vi "_Enqueue JKISMQ.vi"(8 "Error in":errorcluster caption="Error in (no error)", 10 "Data":T1, 11 "JKISMQ":T2) -> (0 "Error out":errorcluster, 3 "JKISMQ":T2)   [LabVIEW 2020, in "JKI-State-Machine-Plus.lvlib"]
uses:
  JKI-State-Machine-Plus.lvlib
  _JKISMQ.ctl
  _Cross JKI StateMachine State Data.ctl
  _Cross JKI StateMachine State Response.ctl
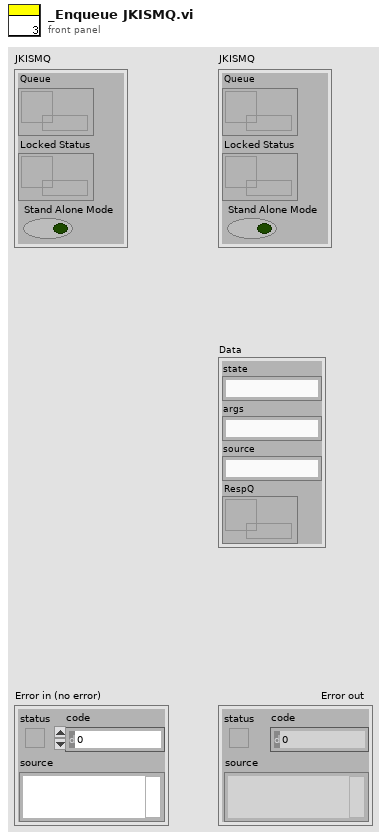
[diagram p1: front panel]
types:
  T1 = typedef "JKI-State-Machine-Plus.lvlib/_Cross JKI StateMachine State Data.ctl" = cluster{"state":string, "args":string, "source":string, "RespQ":refnum<queue>}
  T2 = typedef "JKI-State-Machine-Plus.lvlib/_JKISMQ.ctl" = cluster{"Queue":refnum<queue>, "Locked Status":refnum<data-value>, "Stand Alone Mode":bool}
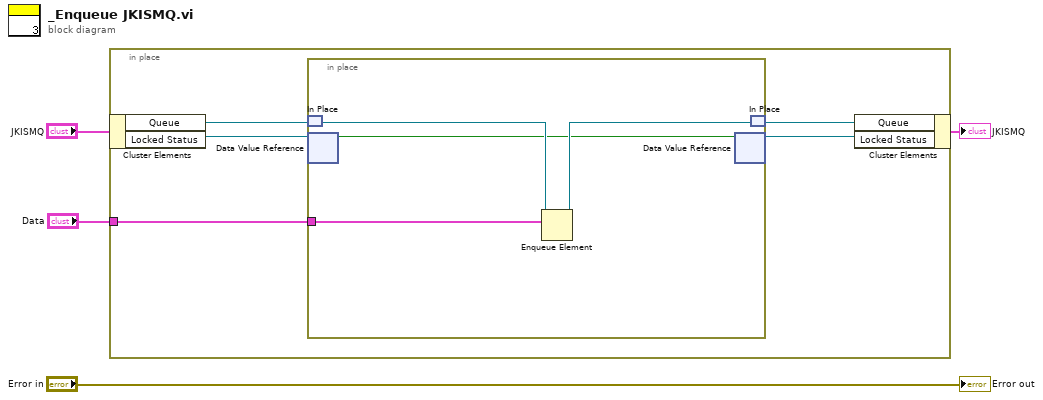
[diagram p0: block diagram]
diagram:
  n1 = in-place "In Place Element Structure" {
    in-place-border: "Data" -> [w5]
    n2 = in-place-cluster #1("JKISMQ") -> ("Queue"=w9:refnum<queue>, "Locked Status"=w7:refnum<data-value>)
    n3 = in-place {
      in-place-border: w5 -> [w10]
      n4 = in-place-match #2(w9) -> (w12:refnum<queue>)
      n5 = in-place-dvr #3(w7) -> (w11:bool)  [unwired: 1 out]
      n6 = Enqueue Element(queue=w12, element=w10) -> (queue out=w13:refnum<queue>)  [unwired: 2 in, 2 out]
      n7 = in-place-dvr #3(w11) -> (w6:refnum<data-value>)  [unwired: 1 out]
      n8 = in-place-match #2(w13) -> (w8:refnum<queue>)
    }
    n9 = in-place-cluster #1("Queue"=w8, "Locked Status"=w6) -> (→"JKISMQ":T2)
  }
  "Error out" <- "Error in"
